vi "Write Denuded.vi"(8 "error in (no error)":errorcluster, 10 "Denuded":bool, 11 "ePAS Cell Data in":refnum<class "ePAS Cell Data.lvclass">=refnum) -> (0 "error out":errorcluster, 3 "ePAS Cell Data out":refnum<class "ePAS Cell Data.lvclass">)   [LabVIEW 2014, in "ePAS Cell Data.lvclass"]
uses:
  ePAS Cell Data.lvclass
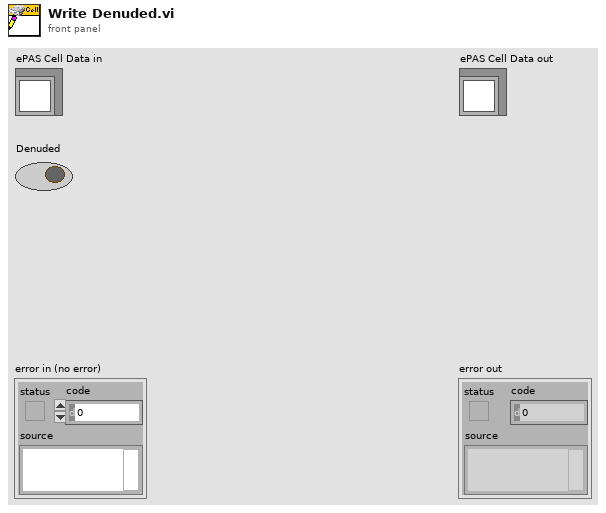
[diagram p1: front panel]
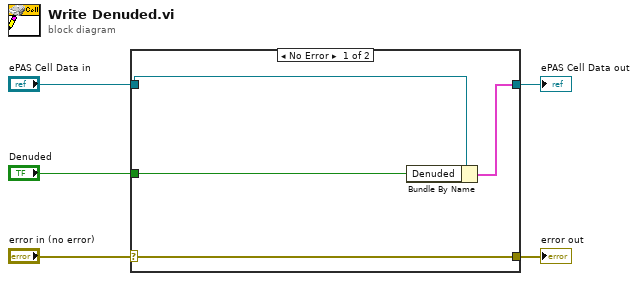
[diagram p0: block diagram]
diagram:
  n1 = case shown="No Error" "error in (no error)" {
    selector: "error in (no error)" -> [w9 w10]
    tunnel: [w9 w10] -> w4
    tunnel: [w7 w11] -> w2
    tunnel: "ePAS Cell Data in" -> [w8 w11]
    tunnel: "Denuded" -> [w6 _]
    frame No Error {
      n2 = Bundle By Name(cluster=w8, "Denuded"=w6) -> (w7:cluster{})
    }
    frame Error {
    }
  }
  "error out" <- w4
  "ePAS Cell Data out" <- w2
